vi "Scale.vi"(8 "error in":errorcluster, 10 "Input":variant, 11 "Scalar Scaling Strategy in":refnum<class "Scalar Scaling Strategy.lvclass">) -> (0 "error out":errorcluster, 2 "Output":variant, 3 "Scalar Scaling Strategy out":refnum<class "Scalar Scaling Strategy.lvclass">)   [LabVIEW 2024, in "HAL.lvlib" / "Scalar Scaling Strategy.lvclass"]
uses:
  Scalar Scaling Strategy.lvclass
  Scalar Scaling Strategy.lvclass/Scalar Scaling Strategy.ctl
  <userlib>/_OpenG.lib/lvdata/lvdata.llb/openg_variant.lvlib
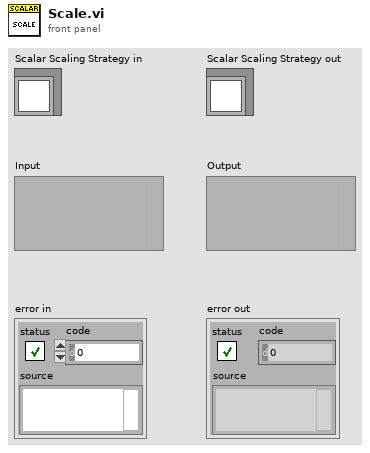
[diagram p1: front panel]
types:
  T1 = typedef "openg_variant.lvlib/Type Descriptor Enumeration__ogtk.ctl" = enum8{"<Null>", "I8", "I16", "I32", "I64", "U8", "U16", "U32", "U64", "SGL", "DBL", "EXT", "CSG", "CDB", "CXT", "0x0F", "0x10", "0x11", "0x12", "0x13", "0x14", "Enum U8", "Enum U16", "Enum U32", "Enum U64", "SGL PQ", "DBL PQ", "EXT PQ", "CSG PQ", "CDB PQ", "CXT PQ", "0x1F", "0x20", "Boolean", "0x22", "0x23", "0x24", "0x25", "0x26", "0x27", "0x28", "0x29", "0x2A", "0x2B", "0x2C", "0x2D", "0x2E", "0x2F", "String", "0x31", "Path", "Pict", "0x34", "0x35", "0x36", "DAQ", "0x38", "0x39", "0x3A", "0x3B", "0x3C", "0x3D", "0x3E", "0x3F", "Array", "0x41", "0x42", "0x43", "0x44", "0x45", "0x46", "0x47", "0x48", "0x49", "0x4A", "0x4B", "0x4C", "0x4D", "0x4E", "0x4F", "Cluster", "0x51", "0x52", "Variant", "Waveform", "0x55", "0x56", "0x57", "0x58", "0x59", "0x5A", "0x5B", "0x5C", "0x5D", "0x5E", "Fixed Point", "0x60", "0x61", "0x62", "0x63", "0x64", "0x65", "0x66", "0x67", "0x68", "0x69", "0x6A", "0x6B", "0x6C", "0x6D", "0x6E", "0x6F", "Refnum", "0x71", "0x72", "Set Collection", "Map Collection"}
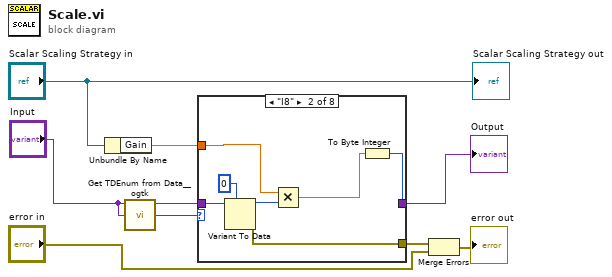
[diagram p0: block diagram]
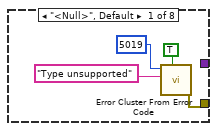
[diagram p2: hidden frame]
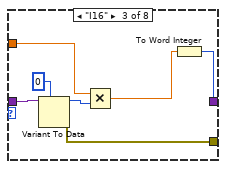
[diagram p3: hidden frame]
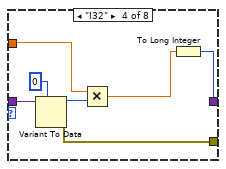
[diagram p4: hidden frame]
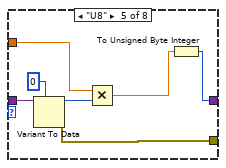
[diagram p5: hidden frame]
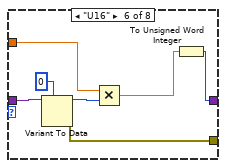
[diagram p6: hidden frame]
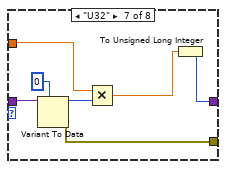
[diagram p7: hidden frame]
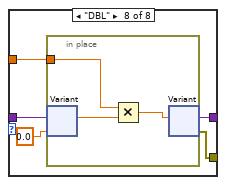
[diagram p8: hidden frame]
diagram:
  n1 = Unbundle By Name("Scalar Scaling Strategy in") -> ("Gain"=w7:dbl)
  n2 = call <userlib>:"Get TDEnum from Data__ogtk.vi"("Data"="Input") -> ("Type Descriptor Enumeration"=w4:T1)  [unwired: 4 in]
  n3 = case shown="\"I8\"" w4 {
    tunnel: [w12 w15 w22 w30 w36 w43 w50 w56] -> w5
    tunnel: [_ w17 w24 w31 w37 w44 w51 w55] -> w6
    tunnel: w7 -> [_ w16 w23 w32 w38 w45 w52 w59]
    tunnel: "Input" -> [_ w13 w20 w27 w34 w41 w48 w58]
    frame "<Null>", Default {
      n4 = call <vilib>:"Error Cluster From Error Code.vi"("show call chain? (False)"=TRUE, "error message (\"\")"="Type unsupported" ("error message (\"\")"), "error code (0)"=5019) -> ("error out"=w12:errorcluster)  [unwired: 6 in]
    }
    frame "I8" {
      n5 = Variant To Data(type=i8 0, Variant=w13) -> (data=w18:i8, error out=w15:errorcluster)  [unwired: 1 in]
      n6 = Multiply(x=w16, y=w18) -> (x*y=w14:dbl)
      n7 = To Byte Integer(number=w14) -> (8bit integer=w17:i8)
    }
    frame "I16" {
      n8 = Variant To Data(type=i16 0, Variant=w20) -> (data=w25:i16, error out=w22:errorcluster)  [unwired: 1 in]
      n9 = Multiply(x=w23, y=w25) -> (x*y=w21:dbl)
      n10 = To Word Integer(number=w21) -> (16bit integer=w24:i16)
    }
    frame "I32" {
      n11 = Variant To Data(type=0, Variant=w27) -> (data=w29:i32, error out=w30:errorcluster)  [unwired: 1 in]
      n12 = Multiply(x=w32, y=w29) -> (x*y=w28:dbl)
      n13 = To Long Integer(number=w28) -> (32bit integer=w31:i32)
    }
    frame "U8" {
      n14 = Variant To Data(type=u8 0, Variant=w34) -> (data=w39:u8, error out=w36:errorcluster)  [unwired: 1 in]
      n15 = Multiply(x=w38, y=w39) -> (x*y=w35:dbl)
      n16 = To Unsigned Byte Integer(number=w35) -> (unsigned 8bit integer=w37:u8)
    }
    frame "U16" {
      n17 = Variant To Data(type=u16 0, Variant=w41) -> (data=w46:u16, error out=w43:errorcluster)  [unwired: 1 in]
      n18 = Multiply(x=w45, y=w46) -> (x*y=w42:dbl)
      n19 = To Unsigned Word Integer(number=w42) -> (unsigned 16bit integer=w44:u16)
    }
    frame "U32" {
      n20 = Variant To Data(type=u32 0, Variant=w48) -> (data=w53:u32, error out=w50:errorcluster)  [unwired: 1 in]
      n21 = Multiply(x=w52, y=w53) -> (x*y=w49:dbl)
      n22 = To Unsigned Long Integer(number=w49) -> (unsigned 32bit integer=w51:u32)
    }
    frame "DBL" {
      n23 = in-place {
        in-place-border: w59 -> [w62]
        n24 = in-place-variant #1(w58, 0.0) -> (w61:dbl)  [unwired: 1 out]
        n25 = Multiply(x=w62, y=w61) -> (x*y=w60:dbl)
        n26 = in-place-variant #1(w60) -> (w55:variant, w56:errorcluster)
      }
    }
  }
  "Output" <- w6
  n27 = Merge Errors(w5, "error in") -> (→"error out":errorcluster)
  "Scalar Scaling Strategy out" <- "Scalar Scaling Strategy in"
